vi "Persistent Position.vi"(6 "VI ID":string caption="VI ID (<VI Name>)", 8 "Error In":errorcluster, 9 "Default Position":refnum<class "Window Position.lvclass"> caption="Default Position (Center Top Level)", 10 "Path":path caption="Path (<User App Data>/<App Name>/Window Positions.ini)") -> (0 "Error Out":errorcluster, 3 "Persistent Position out":refnum<class "Window Position.lvclass">)   [LabVIEW 2019, in "Panel.lvlib" / "Persistent Position.lvclass"]
doc: "Persists the VI position to file. If no position information is found in the file, the window will be positioned according to the \"Default Position\" input.\n\n<B>Path:</B> Sets the path to store persistent position information.\n<B>Default Position:</B> Window Position object.\n<b>VI ID:</b> Indexes the position in the file. By default the VI Name is used.\n<B>Error In:</B> Describes error conditions that occur before this node runs.\n\n<B>Persistent Position Out:</B> Persistent Position object.\n<B>Error Out:</B> Contains error information.\n----\nPlease see the following web address for additional documentation and tutorial information:\nhttp://www.mooregoodideas.com/mgi-panel-manager/\n\nAuthor: Derek Trepanier\n\nCopyright (c) 2018, Moore Good Ideas, Inc.\n\nAll rights reserved.\n\nRedistribution and use in source and binary forms, with or without modification, are permitted provided that the following conditions are met:\n\n * Redistributions of source code must retain the above copyright notice, this list of conditions and the following disclaimer.\n * Redistributions in binary form must reproduce the above copyright notice, this list of conditions and the following disclaimer in the documentation and/or other materials provided with the distribution.\n * Neither the name of Moore Good Ideas, Inc. nor the names of its contributors may be used to endorse or promote products derived from this software without specific prior written permission.\n\nTHIS SOFTWARE IS PROVIDED BY THE COPYRIGHT HOLDERS AND CONTRIBUTORS \"AS IS\" AND ANY EXPRESS OR IMPLIED WARRANTIES, INCLUDING, BUT NOT LIMITED TO, THE IMPLIED WARRANTIES OF MERCHANTABILITY AND FITNESS FOR A PARTICULAR PURPOSE ARE DISCLAIMED. IN NO EVENT SHALL THE COPYRIGHT OWNER OR CONTRIBUTORS BE LIABLE FOR ANY DIRECT, INDIRECT, INCIDENTAL, SPECIAL, EXEMPLARY, OR CONSEQUENTIAL DAMAGES (INCLUDING, BUT NOT LIMITED TO, PROCUREMENT OF SUBSTITUTE GOODS OR SERVICES; LOSS OF USE, DATA, OR PROFITS; OR BUSINESS INTERRUPTION) HOWEVER CAUSED AND ON ANY THEORY OF LIABILITY, WHETHER IN CONTRACT, STRICT LIABILITY, OR TORT (INCLUDING NEGLIGENCE OR OTHERWISE) ARISING IN ANY WAY OUT OF THE USE OF THIS SOFTWARE, EVEN IF ADVISED OF THE POSSIBILITY OF SUCH DAMAGE."
uses:
  Persistent Position.lvclass
  Window Position.lvclass
  C:/Users/Public/Documents/Development/Drivers/Source/Utilities/Actor Framework Tools/Panel Manager/Panel/Window Position/Window Position.lvclass
  Persistent Position.lvclass/Persistent Position.ctl
  Reference Position/Ref Top Level/Ref Top Level.lvclass
  <vilib>/Utility/error.llb/Error Cluster From Error Code.vi
  <vilib>/ErrorRing/Error Ring.xnode
  C:/Users/Public/Documents/Development/Drivers/Source/Utilities/Actor Framework Tools/Panel Manager/Panel/Window Position/Reference Position/Reference Position.lvclass
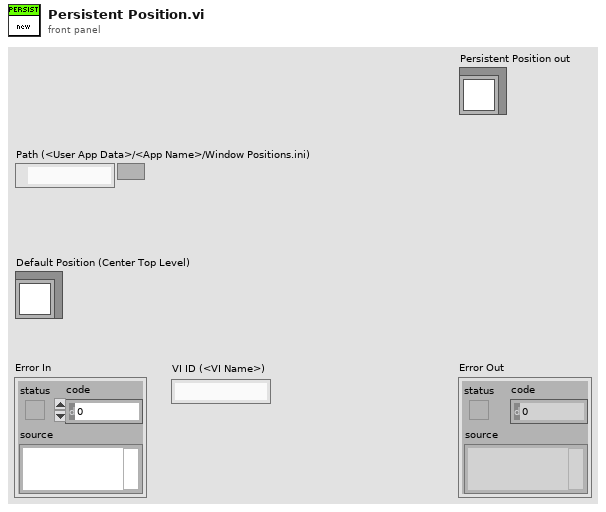
[diagram p1: front panel]
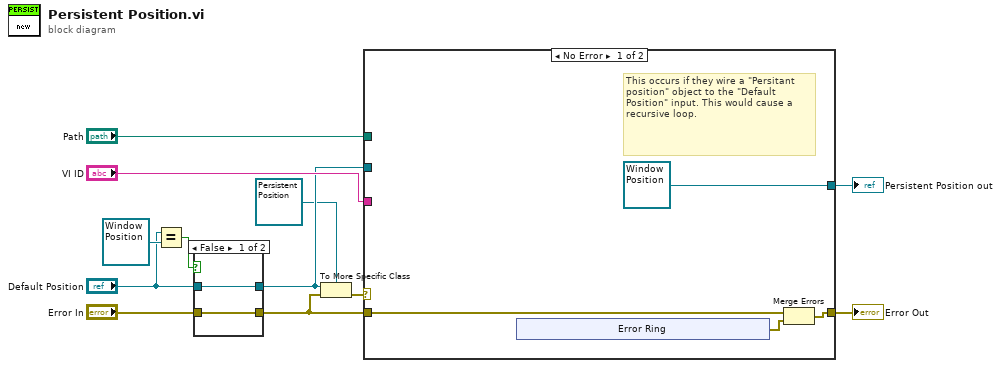
[diagram p0: block diagram]
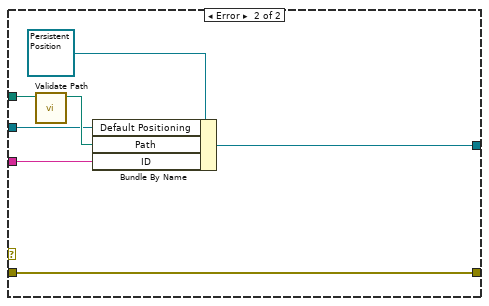
[diagram p2: hidden frame]
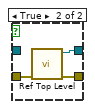
[diagram p3: hidden frame]
diagram:
  n1 = Equal?(x="Default Position", y=refnum<class "Window Position.lvclass"> refnum) -> (x = y?=w10:bool)
  n2 = case shown="False" w10 {
    tunnel: [w14 w17] -> w5
    tunnel: "Default Position" -> [w14 _]
    tunnel: [w13 w16] -> w1
    tunnel: "Error In" -> [w13 w15]
    frame False {
    }
    frame True {
      n3 = call "Ref Top Level.vi"("Error In"=w15) -> ("Error Out"=w16:errorcluster, "Ref Top Level out"=w17:refnum<class "Ref Top Level.lvclass">)  [unwired: 9 in]
    }
  }
  n4 = To More Specific Class(target class=refnum<class "Persistent Position.lvclass"> refnum ("Persistent Position in"), reference=w5, error in=w1) -> (error out=w3:errorcluster)  [unwired: 1 out]
  n5 = case shown="No Error" w3 {
    tunnel: [refnum<class "Window Position.lvclass"> refnum ("Default Positioning") w33] -> w12
    tunnel: "Path" -> [_ w32]
    tunnel: "VI ID" -> [_ w30]
    tunnel: w5 -> [_ w29]
    tunnel: [w19 w27] -> w2
    tunnel: w1 -> [w20 w27]
    frame No Error {
      # "This occurs if they wire a \"Persitant position\" object to the \"Default Position\" input. This would cause a recursive loop."
      n6 = xnode "Error Ring"() -> ("error out"=w18:errorcluster)
      n7 = Merge Errors(w20, w18) -> (w19:errorcluster)
    }
    frame Error {
      n8 = call "Validate Path.vi"("Path in"=w32) -> ("Path out"=w31:path)  [unwired: 10 in]
      n9 = Bundle By Name(cluster=refnum<class "Persistent Position.lvclass"> refnum ("Persistent Position in"), "Default Positioning"=w29, "Path"=w31, "ID"=w30) -> (w33:refnum<class "Persistent Position.lvclass">)
    }
  }
  "Error Out" <- w2
  "Persistent Position out" <- w12
